vi "Close.vi"(7 "Abort (F)":bool, 8 "error in (no error)":errorcluster, 11 "Queue in":refnum<class "Lossless.lvclass">) -> (0 "error out":errorcluster)   [LabVIEW 2022 SP3, in "Enclave.lvlib" / "Lossless.lvclass"]
uses:
  Lossless.lvclass
  Lossless.lvclass/Lossless.ctl
  Enclave/Enclave.lvclass
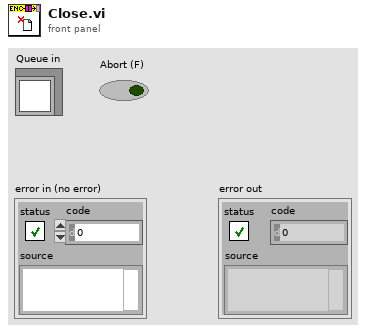
[diagram p1: front panel]
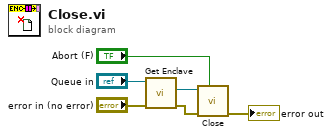
[diagram p0: block diagram]
diagram:
  n1 = call "Get Enclave.vi"("error in (no error)"="error in (no error)", "Lossless in"="Queue in") -> ("error out"=w2:errorcluster, "Enclave"=w4:refnum<class "Enclave.lvclass">)  [unwired: 7 in, 1 out]
  n2 = call "Close.vi"("Abort (F)"="Abort (F)", "error in (no error)"=w2, "Enclave in"=w4) -> ("error out"=→"error out":errorcluster)  [unwired: 8 in]
